vi "add new tag.vi"(8 "error in":errorcluster, 11 "engine configuration in":refnum<class "engine configuration.lvclass">) -> (0 "error out":errorcluster, 3 "engine configuration out":refnum<class "engine configuration.lvclass">)   [LabVIEW 2013, in "PL Framework Configuration Tool.lvlib" / "EngineTags.lvclass"]
uses:
  EngineTags.lvclass
  <vilib>/NI/Module Execution Interface/Engine Configuration/engine configuration.lvclass
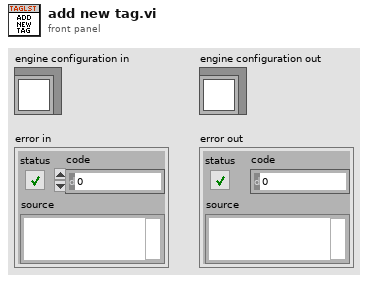
[diagram p1: front panel]
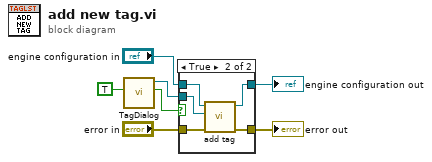
[diagram p0: block diagram]
diagram:
  n1 = call "TagDialog.vi"("new?"=TRUE) -> ("valid?"=w2:bool, "new tag"=w3:refnum<class "tag descriptor.lvclass">)  [unwired: 7 in, 2 out]
  n2 = case shown="True" w2 {
    tunnel: w3 -> [_ w14]
    tunnel: "engine configuration in" -> [w9 w13]
    tunnel: [w9 w12] -> w5
    tunnel: "error in" -> [w8 w11]
    tunnel: [w8 w10] -> w7
    frame False {
    }
    frame True {
      n3 = call <vilib>:"add tag.vi"("error in"=w11, "tag descriptor"=w14, "engine configuration in"=w13) -> ("error out"=w10:errorcluster, "engine configuration out"=w12:refnum<class "engine configuration.lvclass">)  [unwired: 7 in]
    }
  }
  "error out" <- w7
  "engine configuration out" <- w5
